vi "Receive.vi"(6 "clear_timeout_error (f)":bool, 7 "mode (standard)":T1(ring), 8 "error in (no error)":errorcluster, 10 "bufsize (0)":u32, 11 "Socket.TCP in":refnum<class "Socket.TCP.lvclass">) -> (0 "error out":errorcluster, 1 "bytes_read":i32, 2 "data_out":string, 3 "Socket.TCP out":refnum<class "Socket.TCP.lvclass">)   [LabVIEW 2014, in "Socket.lvlib" / "Socket.TCP.lvclass"]
doc: "socket.tcp.Receive (mode, bufsize, [clear_timeout_error]) Waits for the timeout period in ms and returns bytes received or timeout error.\n\nenum mode\n Standard: Waits until all bytes in bufsize arrive or until timeout. If timeout occurs, returns the bytes read so far and reports timeout error.\n Buffered: Waits until all bytes in bufsize arrive or until timeout. If timeout occurs, returns no bytes and reports timeout error\n CRLF: Waits until all bytes in bufsize arrive or until a carriage return (CR) followed by a linefeed (LF) or until timeout. Returns all bytes including the CR and LF. If timeout occurs before CRLF, returns no bytes and a timeout error.\n Immediate: Waits until any bytes in bufsize arrive. Only reports a timeout errror if no bytes arrive.\n\nu32 bufsize is the amount of bytes the receiver will wait for as determined by mode. If bufsize = 0, the incoming bytes are assumed to be a TCP packet and the first two bytes will be used to determine the size of the following packet to be received.\n\nbool clear_timeout_error optional input to clear the timeout error before exiting the method. This is used when looping receive to check for loop exit conditions."
uses:
  Socket.TCP.lvclass
  Socket.TCP.lvclass/Socket.TCP.ctl
  Socket.Base/Socket.Base.lvclass/Socket.Base.ctl
  Accessors/Read tcp _refnum.vi
  Socket.Base/Accessors/Read timeout.vi
panel:
  # "If bufsize is 0, a TCP packet is assumed and the first two bytes will be used as the packet size."
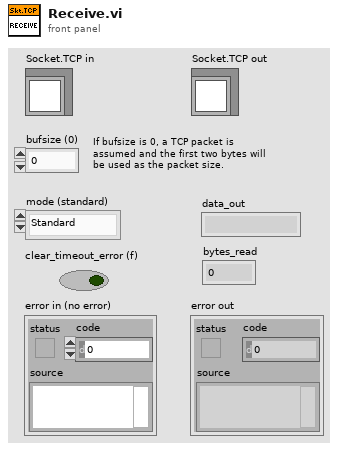
[diagram p1: front panel]
types:
  T1 = enum16{"Standard", "Buffered", "CRLF", "Immediate"}
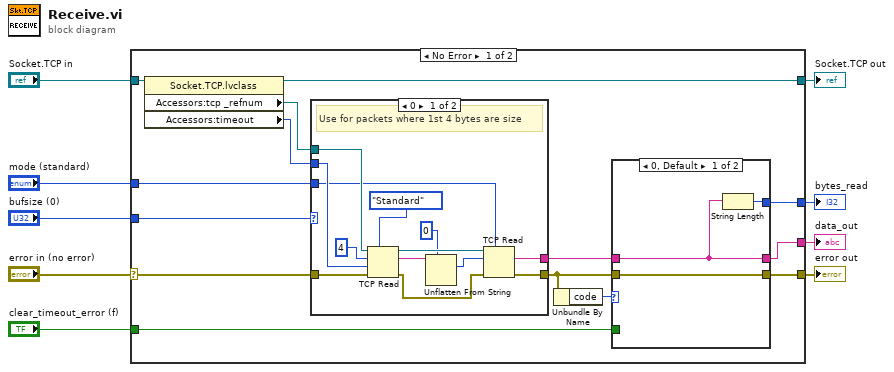
[diagram p0: block diagram]
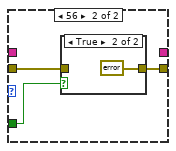
[diagram p2: hidden frame]
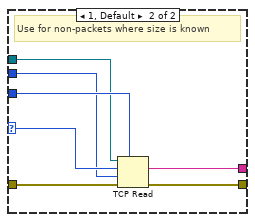
[diagram p4: hidden frame]
diagram:
  n1 = case shown="No Error" "error in (no error)" {
    selector: "error in (no error)" -> [w17 w53]
    tunnel: [w16 w53] -> w8
    tunnel: [w22 w52] -> w6
    tunnel: "Socket.TCP in" -> [w23 w52]
    tunnel: "mode (standard)" -> [w21 _]
    tunnel: "bufsize (0)" -> [w20 _]
    tunnel: "clear_timeout_error (f)" -> [w15 _]
    tunnel: [w11 _] -> w2
    tunnel: [w10 _] -> w1
    frame No Error {
      n2 = property class="Socket.TCP.lvclass"(reference=w23) -> (reference out=w22:refnum<class "Socket.TCP.lvclass">, "Accessors:tcp _refnum"=w18:refnum<k5>, "Accessors:timeout"=w19:i32)  [unwired: 1 in, 1 out]
      n3 = case shown="0" w20 {
        selector: w20 -> [_ w46]
        tunnel: w21 -> [w38 w48]
        tunnel: w19 -> [w39 w45]
        tunnel: w18 -> [w40 w47]
        tunnel: w17 -> [w37 w51]
        tunnel: [w36 w50] -> w13
        tunnel: [w35 w49] -> w14
        frame 0 {
          # "Use for packets where 1st 4 bytes are size"
          n4 = TCP Read(connection ID=w40, bytes to read=4, error in (no error)=w37, 7:T1."Standard" ("mode (standard)"), 9:w39) -> (connection ID out=w42:refnum<k5>, data out=w33:string, error out=w44:errorcluster)
          n5 = Unflatten From String(type=u32 0 ("default (0 I32)"), binary string=w33) -> (value=w32:u32)  [unwired: 3 in, 2 out]
          n6 = TCP Read(connection ID=w42, bytes to read=w32, error in (no error)=w44, 7:w38) -> (data out=w35:string, error out=w36:errorcluster)  [unwired: 1 in, 1 out]
        }
        frame 1, Default {
          # "Use for non-packets where size is known"
          n7 = TCP Read(connection ID=w47, bytes to read=w46, error in (no error)=w51, 7:w48, 9:w45) -> (data out=w49:string, error out=w50:errorcluster)  [unwired: 1 out]
        }
      }
      n8 = Unbundle By Name(w13) -> ("code"=w12:i32)
      n9 = case shown="0, Default" w12 {
        tunnel: w13 -> [w26 w29]
        tunnel: [w26 w28] -> w16
        tunnel: w14 -> [w24 _]
        tunnel: [w24 _] -> w10
        tunnel: [w25 _] -> w11
        tunnel: w15 -> [_ w27]
        frame 0, Default {
          n10 = String Length(string=w24) -> (length=w25:i32)
        }
        frame 56 {
          n11 = case shown="True" w27 {
            tunnel: w29 -> [w30 _]
            tunnel: [w30 errorcluster {"status"=FALSE, "code"=0, "source"=""} ("error constant")] -> w28
            frame False {
            }
            frame True {
            }
          }
        }
      }
    }
    frame Error {
    }
  }
  "error out" <- w8
  "Socket.TCP out" <- w6
  "bytes_read" <- w2
  "data_out" <- w1
